vi "RequestDestroy.vi"(8 "ErrorIn":errorcluster, 11 "ReferenceIn":refnum<class "UserManager.lvclass">) -> (0 "ErrorOut":errorcluster, 3 "ReferenceOut":refnum<class "UserManager.lvclass">)   [LabVIEW 2021, in "UserMananger.lvlib" / "UserManager.lvclass"]
uses:
  UserManager.lvclass
  3fbc1877-3ae8-4aff-a423-cebf9be5a0b1.vi
  MainGUIRepository.vi
  UserManager.lvclass/UserManager.ctl
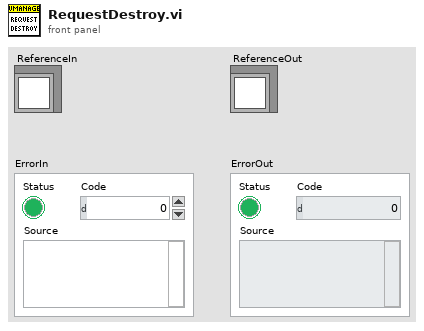
[diagram p1: front panel]
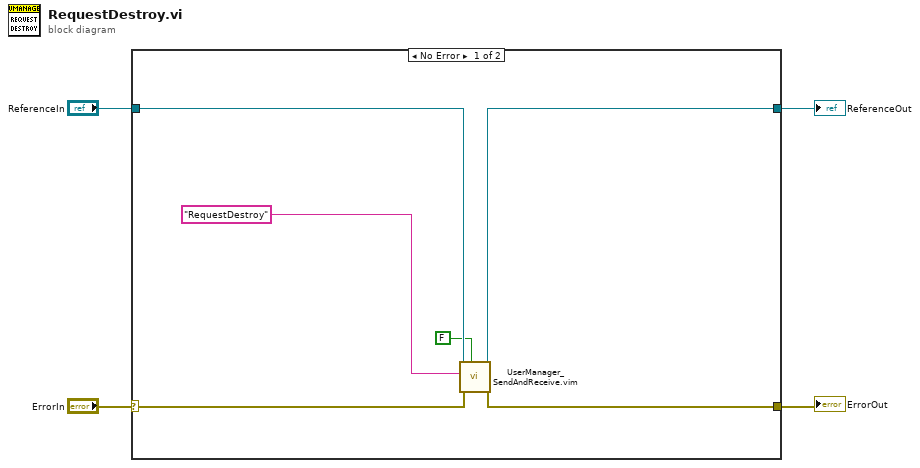
[diagram p0: block diagram]
diagram:
  n1 = case shown="No Error" "ErrorIn" {
    selector: "ErrorIn" -> [w10 w12]
    tunnel: [w9 w12] -> w3
    tunnel: [w7 w11] -> w1
    tunnel: "ReferenceIn" -> [w8 w11]
    frame No Error {
      n2 = call "UserManager_SendAndReceive.vim"("ShouldWeWaitForResponse"=FALSE, "error in (no error)"=w10, "Command"="RequestDestroy", "reference in"=w8) -> ("error out"=w9:errorcluster, "reference out"=w7:refnum<class "UserManager.lvclass">)  [unwired: 5 in, 1 out]
    }
    frame Error {
    }
  }
  "ErrorOut" <- w3
  "ReferenceOut" <- w1
